vi "Set_Picture.vi"(8 "error in (no error)":errorcluster caption="entrée d'erreur (pas d'erreur)", 10 "Picture":picture, 11 "Class Popup Operator_Validation (Default) en entrée":refnum<class "Class Popup Operator_Validation (Virtual).lvclass">) -> (0 "error out":errorcluster caption="sortie d'erreur", 3 "Class Popup Operator_Validation (Default) en sortie":refnum<class "Class Popup Operator_Validation (Virtual).lvclass">)   [LabVIEW 2020, in "Library Instrument & Equipement.lvlib" / "Library Popup.lvlib" / "Class Popup Operator_Validation (Virtual).lvclass"]
uses:
  Class Popup Operator_Validation (Virtual).lvclass
  Class Popup Operator_Validation (Virtual).lvclass/Class Popup Operator_Validation (Virtual).ctl
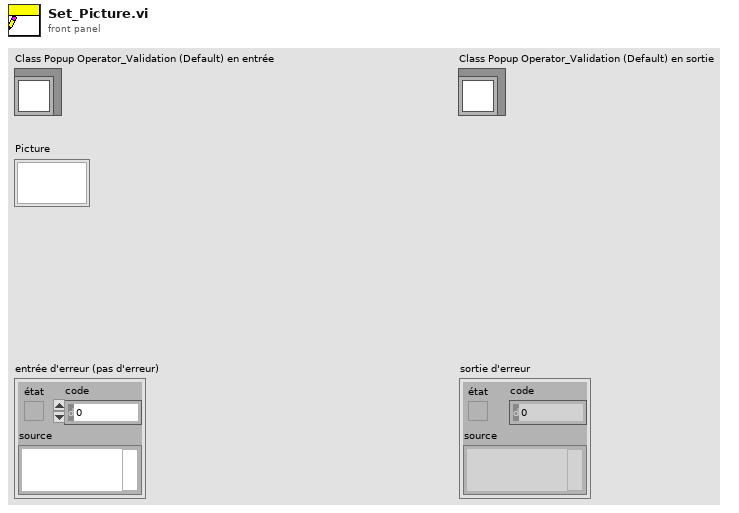
[diagram p1: front panel]
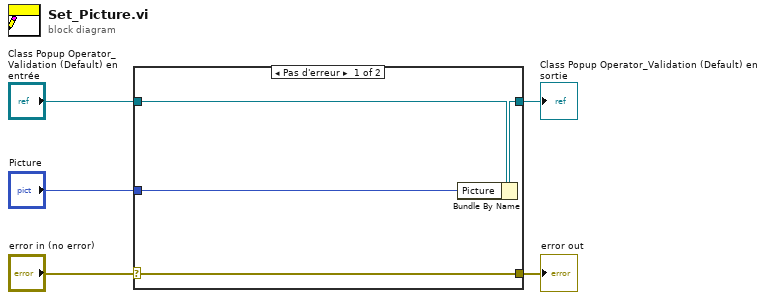
[diagram p0: block diagram]
diagram:
  n1 = case shown="Pas d'erreur" "error in (no error)" {
    selector: "error in (no error)" -> [w9 w10]
    tunnel: [w9 w10] -> w4
    tunnel: [w7 w11] -> w2
    tunnel: "Class Popup Operator_Validation (Default) en entrée" -> [w8 w11]
    tunnel: "Picture" -> [w6 _]
    frame No Error {
      n2 = Bundle By Name(cluster=w8, "Picture"=w6) -> (w7:refnum<class "Class Popup Operator_Validation (Virtual).lvclass">)
    }
    frame Error {
    }
  }
  "error out" <- w4
  "Class Popup Operator_Validation (Default) en sortie" <- w2
